vi "_Connect References to Build Array.vi"(8 "error in":errorcluster, 10 "Sources":refnum<vi>[](array[refnum]), 11 "Build Array Node":refnum<vi>) -> (0 "error out":errorcluster, 2 "New Wires":refnum<vi>[](array[refnum]))   [LabVIEW 2020, in "Build Array of References__RCF.lvlib"]
doc: "Connects several references to the inputs of a Build Array primitive."
uses:
  Build Array of References__RCF.lvlib
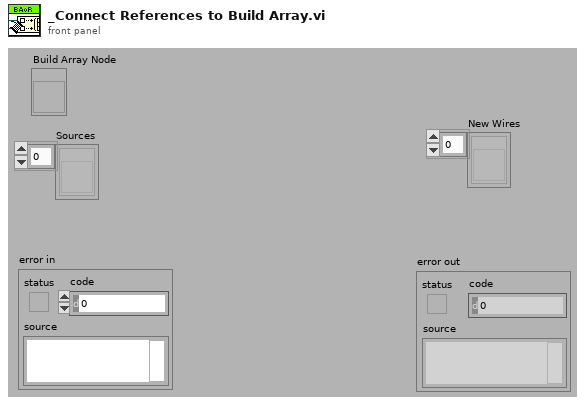
[diagram p1: front panel]
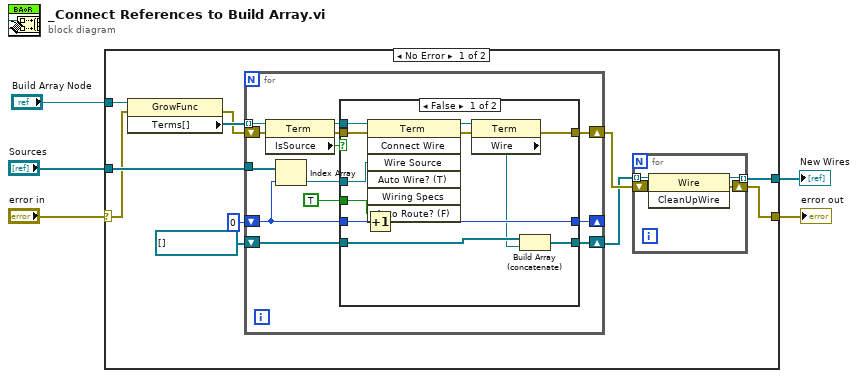
[diagram p0: block diagram]
diagram:
  n1 = case shown="No Error" "error in" {
    selector: "error in" -> [w8 w49]
    tunnel: "Build Array Node" -> [w11 _]
    tunnel: "Sources" -> [w10 _]
    tunnel: [w6 _] -> w3
    tunnel: [w7 w49] -> w1
    frame No Error {
      n2 = property class="GrowFunc"(reference=w11, error in=w8) -> (error out=w14:errorcluster, "Terms[]"=w16:refnum<vi>[])  [unwired: 1 out]
      n3 = for {
        tunnel: w16 -> [w33] mode=indexing
        tunnel: w10 -> [w30]
        shift-right: [w27] -> _
        shift-left: 0 -> [w28]
        shift-right: [w23] -> w12
        shift-left: w14 -> [w26]
        shift-right: [w21] -> w9
        shift-left: refnum<vi>[] [] -> [w22]
        n4 = property class="Term"(reference=w33, error in=w26) -> (reference out=w32:refnum<vi>, error out=w24:errorcluster, "IsSource"=w31:bool)
        n5 = Index Array(array=w30, index=w28) -> (element=w29:refnum<vi>)
        n6 = case shown="False" w31 {
          tunnel: w32 -> [w45 _]
          tunnel: w29 -> [w44 _]
          tunnel: w28 -> [w43 w48]
          tunnel: [w42 w48] -> w27
          tunnel: TRUE ("Auto Route? (F)") -> [w41 _]
          tunnel: w24 -> [w40 w47]
          tunnel: [w34 w47] -> w23
          tunnel: w22 -> [w37 w46]
          tunnel: [w36 w46] -> w21
          frame False {
            n7 = Increment(x=w43) -> (x+1=w42:i32)
            n8 = invoke class="Term" method="Connect Wire"(reference=w45, error in=w40, "Wire Source"=w44, "Auto Route? (F)"=w41) -> (reference out=w39:refnum<vi>, error out=w38:errorcluster)  [unwired: 3 in, 5 out]
            n9 = property class="Term"(reference=w39, error in=w38) -> (error out=w34:errorcluster, "Wire"=w35:refnum<vi>)  [unwired: 1 out]
            n10 = Build Array (concatenate)(w37, w35) -> (w36:refnum<vi>[])
          }
          frame True {
          }
        }
      }
      n11 = for {
        tunnel: w9 -> [w20] mode=indexing
        shift-right: [w18] -> w7
        shift-left: w12 -> [w19]
        tunnel: [w17] -> w6 mode=indexing
        n12 = invoke class="Wire" method="CleanUpWire"(reference=w20, error in=w19) -> (reference out=w17:refnum<vi>, error out=w18:errorcluster)  [unwired: 1 in, 1 out]
      }
    }
    frame Error {
    }
  }
  "New Wires" <- w3
  "error out" <- w1
